vi "Initialize.vi"(8 "error in":errorcluster, 10 "file path":path, 11 "File Logger Interface in":refnum<class "File Type Interface.lvclass">) -> (0 "error out":errorcluster, 3 "File Logger Interface out":refnum<class "File Type Interface.lvclass">)   [LabVIEW 2020, in "File Type Interface.lvclass"]
uses:
  File Type Interface.lvclass
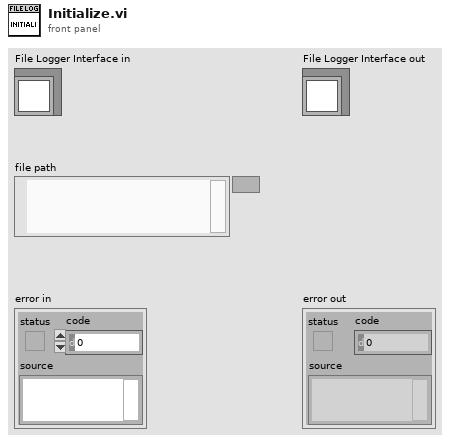
[diagram p1: front panel]
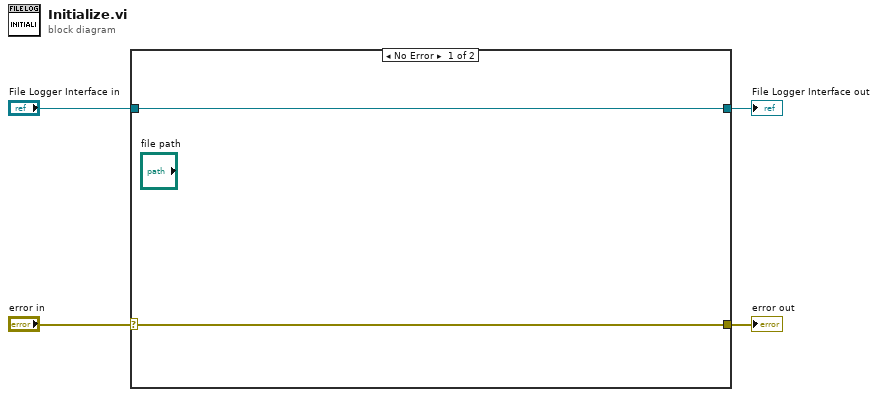
[diagram p0: block diagram]
diagram:
  n1 = case shown="No Error" "error in" {
    selector: "error in" -> [w5 w8]
    tunnel: [w5 w8] -> w3
    tunnel: [w6 w7] -> w1
    tunnel: "File Logger Interface in" -> [w6 w7]
    frame No Error {
    }
    frame Error {
    }
  }
  "error out" <- w3
  "File Logger Interface out" <- w1
